vi "BASE-Main.vi"() -> ()   [LabVIEW 2017]
uses:
  <vilib>/Utility/error.llb/DialogType.ctl
panel:
  out "PLC Simulation ON":bool
  in  "Modify SN":bool
  in  "PRINT":bool
  in  "Torque IO Status":bool
  in  "Ass IO Status":bool
  in  "Recipe":bool
  out "error out":errorcluster
  in  "Logout":bool
  in  "Stop":bool
  in  "Create Login":bool
  in  "Reports":bool
  in  "Start":bool
  out "Time":string
  out "Date":string
  in  "Login":bool
  # "KAPSE SONS ROBOTICS\n& AUTOMATION"
  # "RBC TANK"
types:
  T1 = typedef "DialogType.ctl" = u16
  T2 = enum32{"Invalid", "Standard", "Closed", "Hidden", "Minimized", "Maximized"}
  T3 = enum8{"Enabled", "Disabled", "Disabled and Grayed Out"}
  T4 = enum32{"invalid app kind", "Development System", "Run Time System", "Student Edition", "Embedded LabVIEW", "Evaluation", "Custom"}
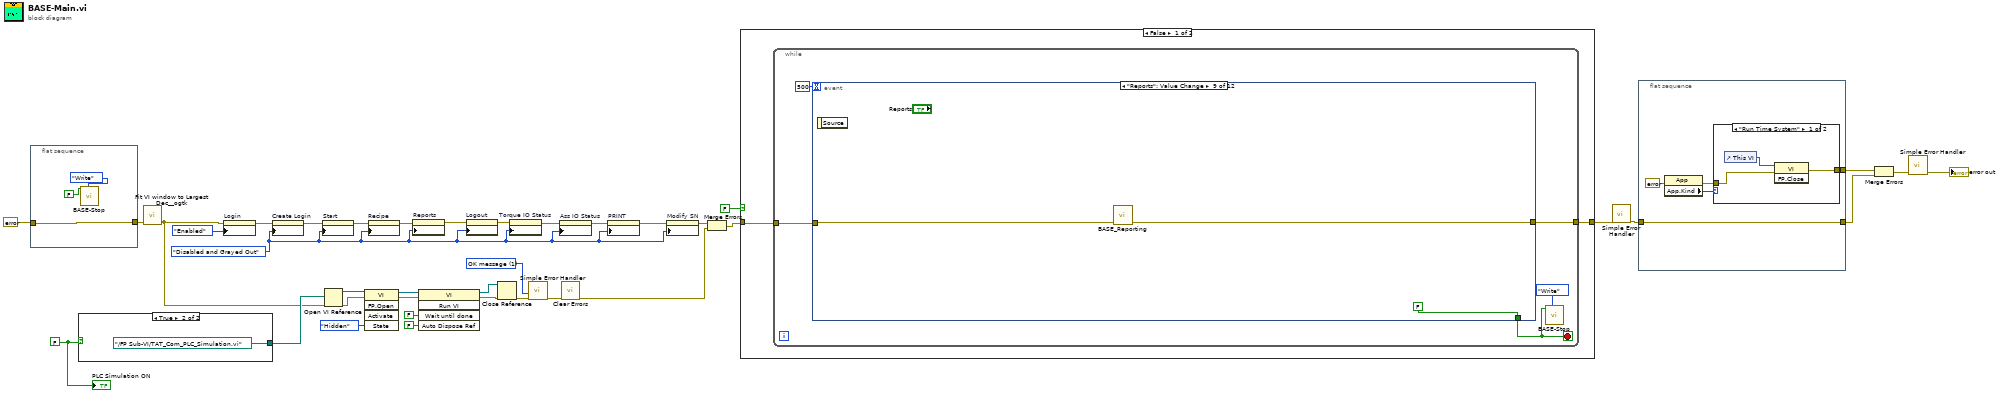
[diagram p0: block diagram]
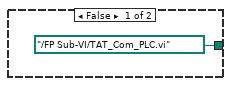
[diagram p2: hidden frame]
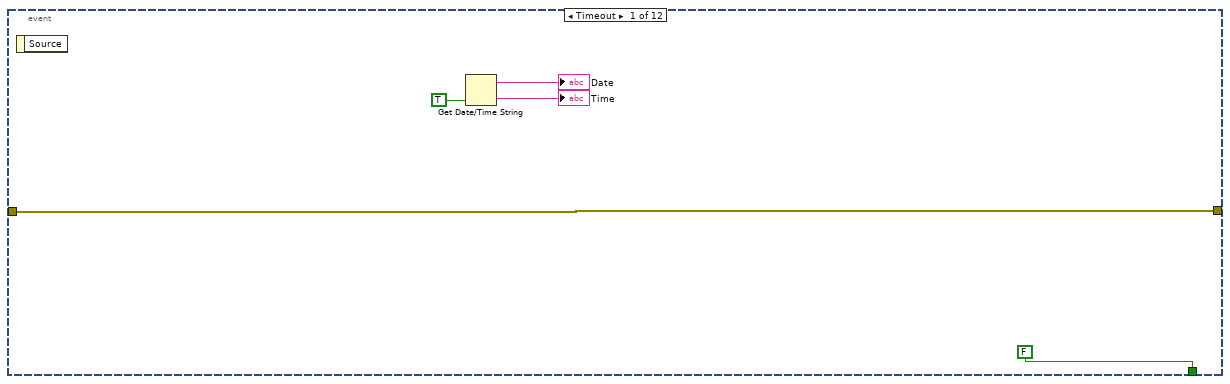
[diagram p4: hidden frame]
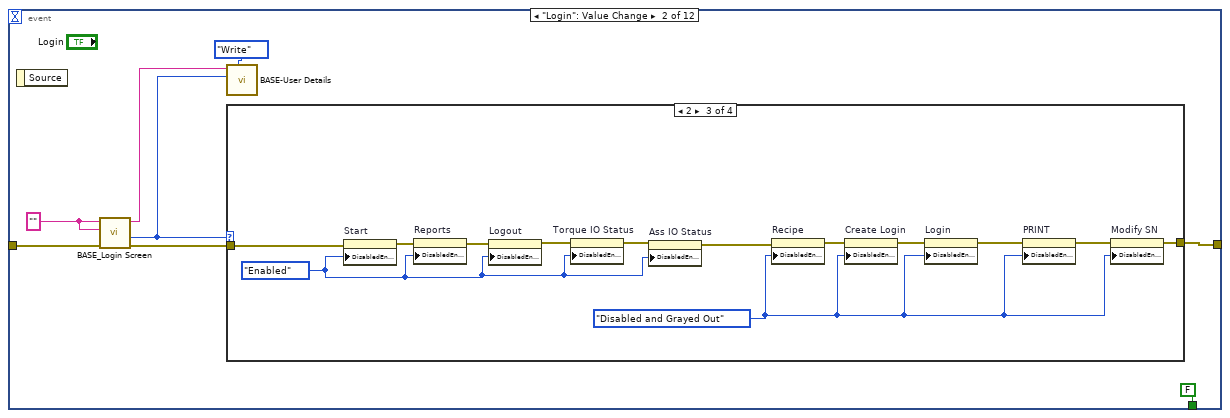
[diagram p5: hidden frame]
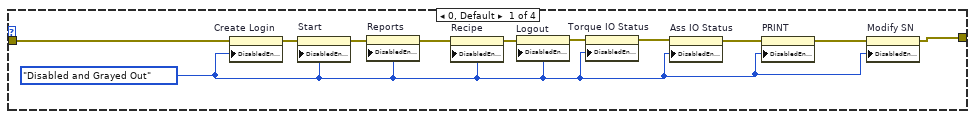
[diagram p6: hidden frame]
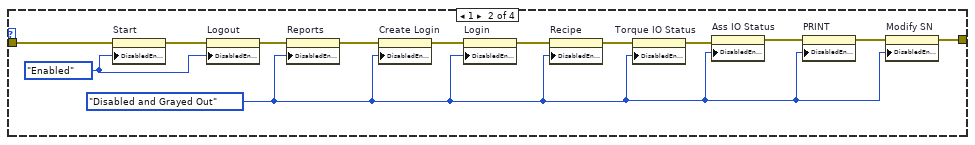
[diagram p7: hidden frame]
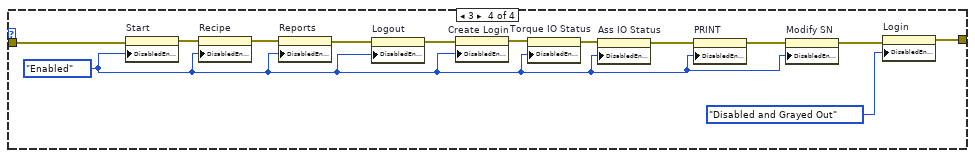
[diagram p8: hidden frame]
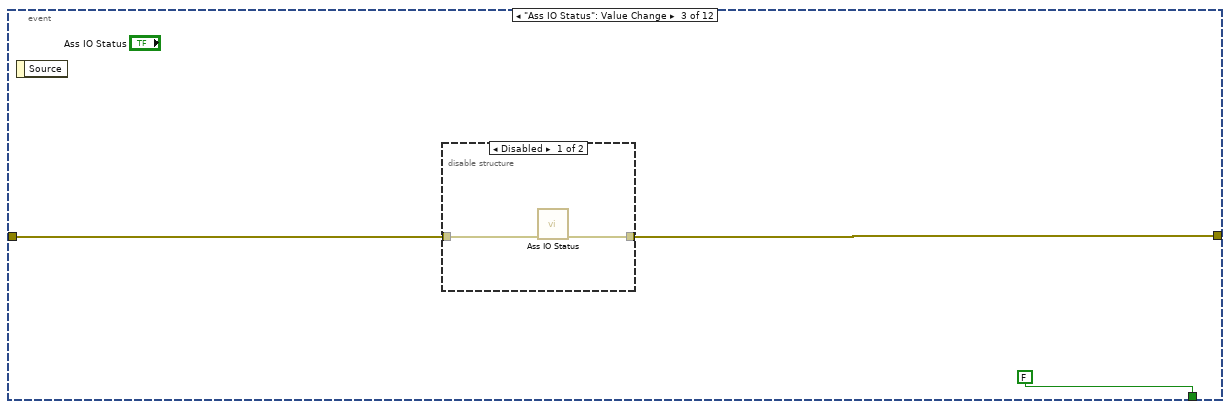
[diagram p9: hidden frame]
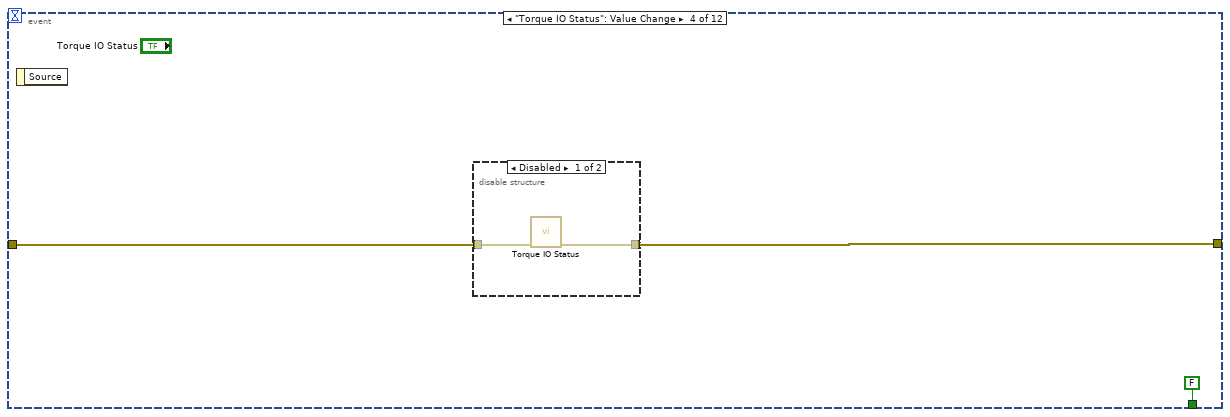
[diagram p11: hidden frame]
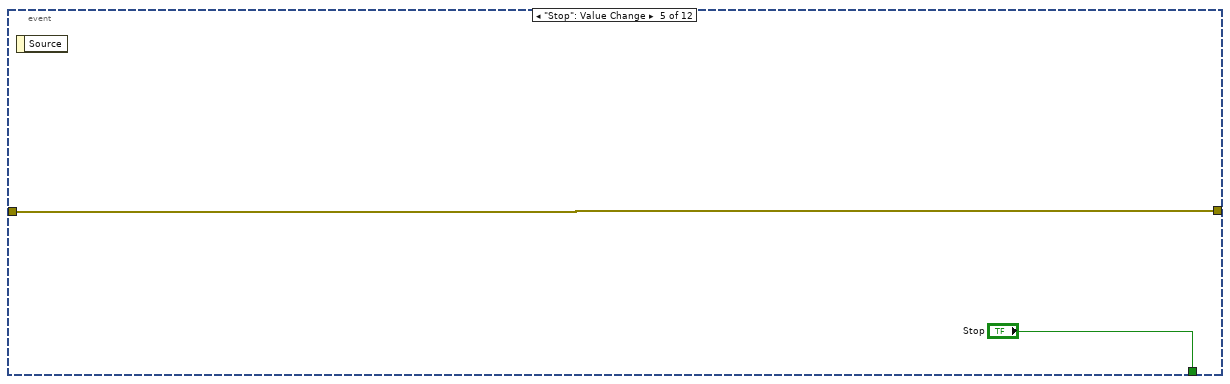
[diagram p13: hidden frame]
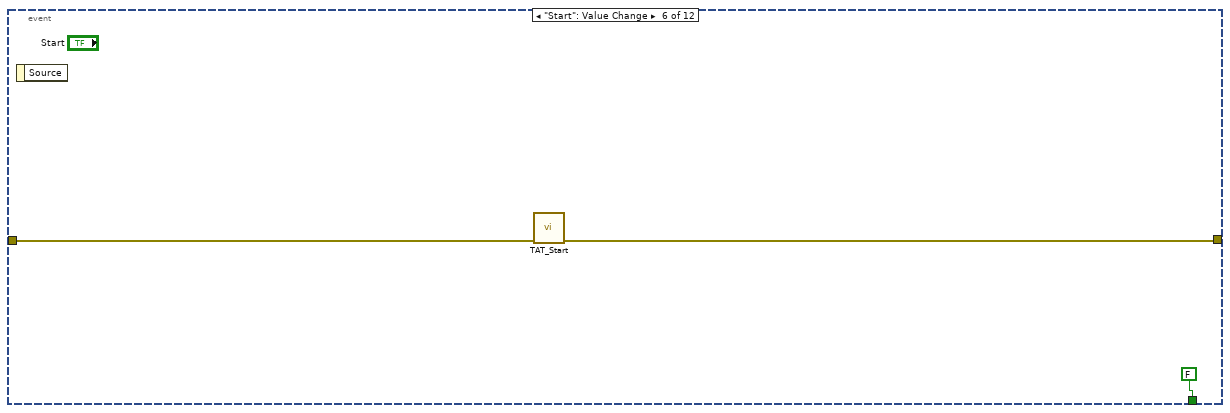
[diagram p14: hidden frame]
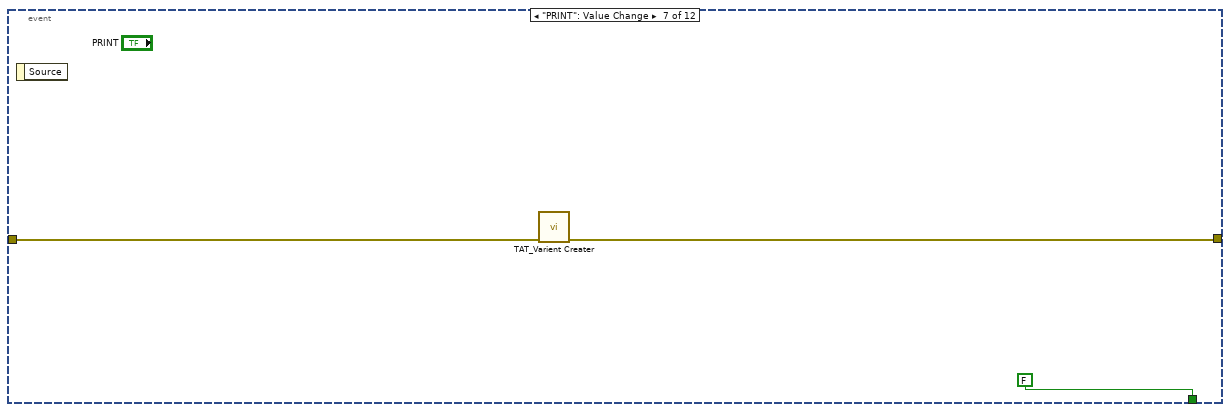
[diagram p15: hidden frame]
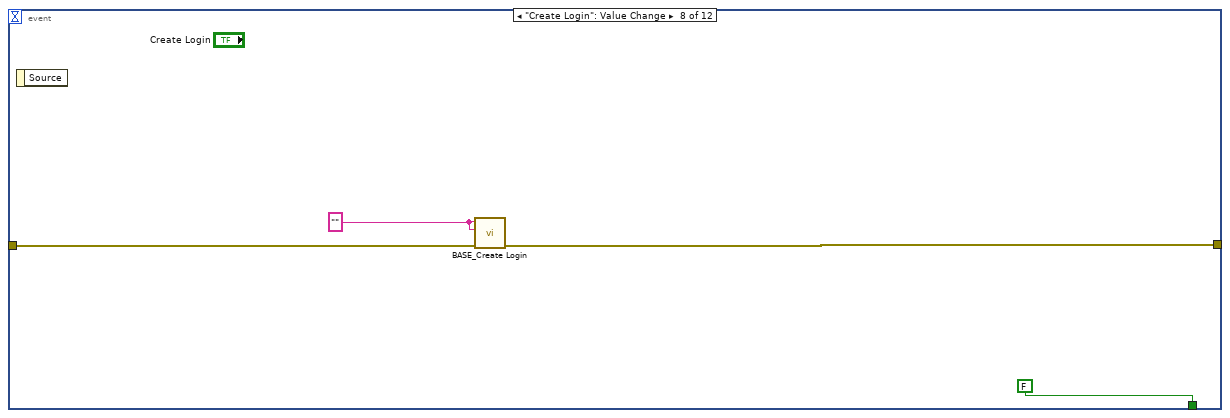
[diagram p16: hidden frame]
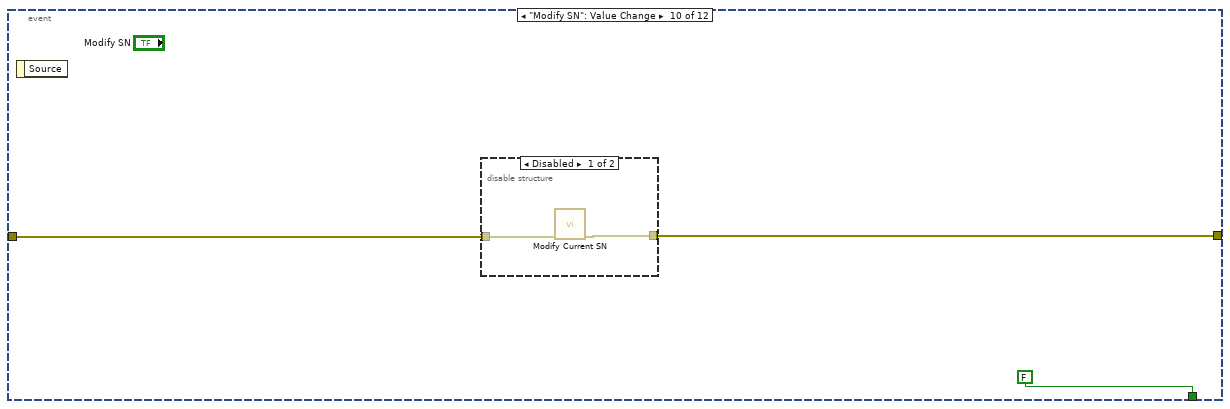
[diagram p17: hidden frame]
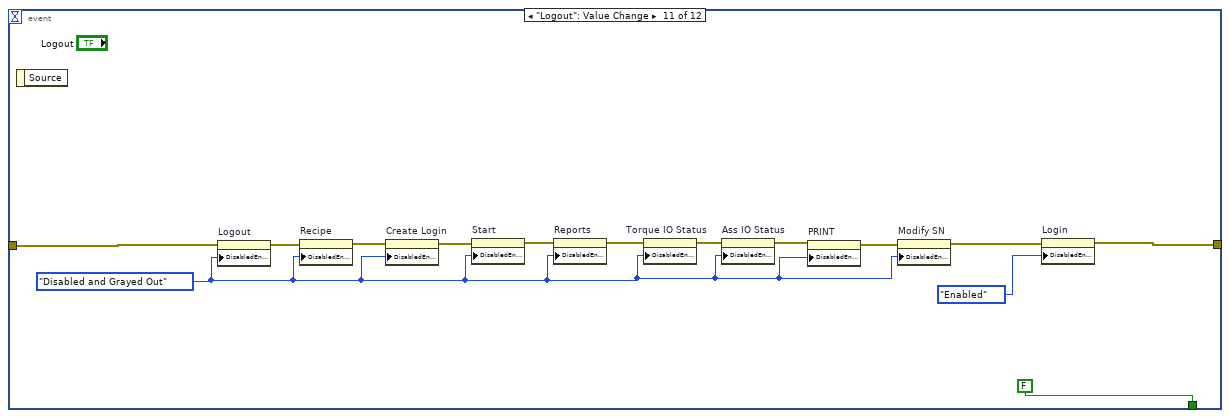
[diagram p19: hidden frame]
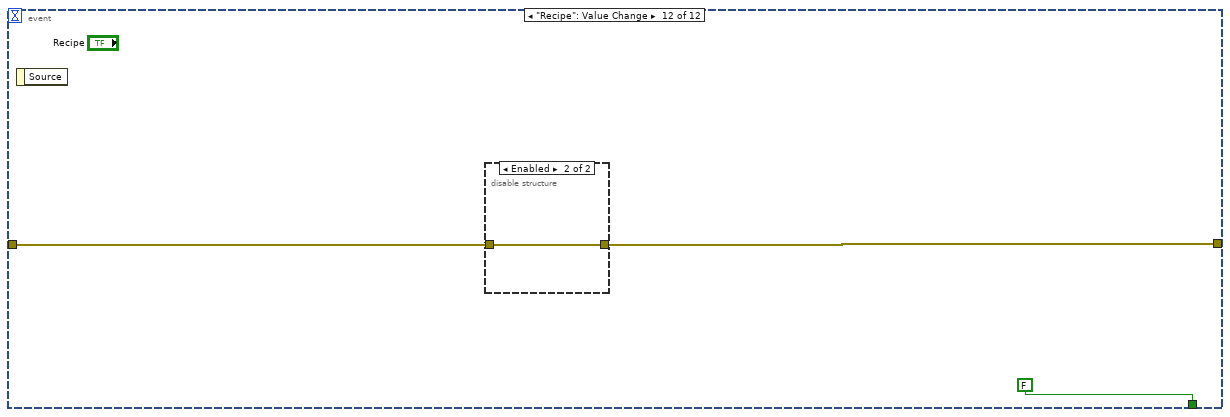
[diagram p20: hidden frame]
diagram:
  w1 = FALSE
  w5 = T1 1 items=["no dialog", "OK message", "continue or stop message", "OK message + warnings", "continue/stop + warnings"] ("type of dialog (OK msg:1)")
  w22 = T3."Disabled and Grayed Out" ("Disabled")
  n1 = flat-sequence {
    tunnel: [w41] -> w20
    tunnel: errorcluster {"status"=FALSE, "code"=0, "source"=""} ("error constant") -> [w41]
    frame #0 {
      n2 = call "BASE-Stop.vi"("Enum"=enum16{"Read", "Write"}."Write", "Stop"=FALSE) -> ()  [unwired: 9 in, 1 out]
    }
  }
  n3 = case shown="True" w1 {
    tunnel: [path "../FP Sub-VI/TAT_Com_PLC.vi" ("vi path") path "../FP Sub-VI/TAT_Com_PLC_Simulation.vi" ("vi path")] -> w11
    frame False {
    }
    frame True {
    }
  }
  n4 = call <userlib>:"Fit VI window to Largest Dec__ogtk.vi"("error in (no error)"=w20) -> ("error out"=w10:errorcluster)  [unwired: 5 in, 1 out]
  n5 = property on="Login" class="Bool"(error in=w10, "DisabledEnum"=T3."Enabled" ("Disabled")) -> (error out=w32:errorcluster)  [unwired: 1 in, 1 out]
  n6 = property on="Create Login" class="Bool"(error in=w32, "DisabledEnum"=w22) -> (error out=w37:errorcluster)  [unwired: 1 in, 1 out]
  n7 = property on="Start" class="Bool"(error in=w37, "DisabledEnum"=w22) -> (error out=w28:errorcluster)  [unwired: 1 in, 1 out]
  n8 = Open VI Reference(vi path=w11, error in (no error)=w10) -> (vi reference=w16:refnum<vi>, error out=w17:errorcluster)  [unwired: 4 in]
  n9 = invoke class="VI" method="FP.Open"(reference=w16, error in=w17, "State"=T2."Hidden") -> (reference out=w19:refnum<vi>, error out=w18:errorcluster)  [unwired: 2 in, 3 out]
  n10 = property on="Recipe" class="Bool"(error in=w28, "DisabledEnum"=w22) -> (error out=w27:errorcluster)  [unwired: 1 in, 1 out]
  n11 = property on="Reports" class="Bool"(error in=w27, "DisabledEnum"=w22) -> (error out=w30:errorcluster)  [unwired: 1 in, 1 out]
  n12 = invoke class="VI" method="Run VI"(reference=w19, error in=w18, "Wait until done"=FALSE ("Wait Until Done"), "Auto Dispose Ref"=FALSE ("Auto Dispose Reference")) -> (reference out=w15:refnum<vi>, error out=w14:errorcluster)  [unwired: 1 in, 3 out]
  n13 = property on="Logout" class="Bool"(error in=w30, "DisabledEnum"=w22) -> (error out=w26:errorcluster)  [unwired: 1 in, 1 out]
  n14 = Close Reference(reference=w15, error in (no error)=w14) -> (error out=w6:errorcluster)
  n15 = property on="Torque IO Status" class="Bool"(error in=w26, "DisabledEnum"=w22) -> (error out=w25:errorcluster)  [unwired: 1 in, 1 out]
  n16 = call <vilib>:"Simple Error Handler.vi"("type of dialog (OK msg:1)"=w5, "error in (no error)"=w6) -> ("error out"=w4:errorcluster)  [unwired: 3 in, 4 out]
  n17 = property on="Ass IO Status" class="Bool"(error in=w25, "DisabledEnum"=w22) -> (error out=w24:errorcluster)  [unwired: 1 in, 1 out]
  n18 = call <vilib>:"Clear Errors.vi"("error in (no error)"=w4) -> ("error out"=w3:errorcluster)  [unwired: 5 in, 1 out]
  n19 = property on="PRINT" class="Bool"(error in=w24, "DisabledEnum"=w22) -> (error out=w23:errorcluster)  [unwired: 1 in, 1 out]
  n20 = property on="Modify SN" class="Bool"(error in=w23, "DisabledEnum"=w22) -> (error out=w8:errorcluster)  [unwired: 1 in, 1 out]
  n21 = Merge Errors(w8, w3) -> (w9:errorcluster)
  n22 = case shown="False" FALSE {
    tunnel: w9 -> [w45 w165]
    tunnel: [w44 w165] -> w38
    frame False {
      n23 = while {
        tunnel: w45 -> [w49]
        tunnel: [w48] -> w44
        stop <- w46 stop-if-true
        n24 = event shown="[8] \"Reports\": Value Change" {
          selector: _ -> [_ _ _ _ _ _ _ _ _ _ _ _]
          dyn-events: _ -> [_ _ _ _ _ _ _ _ _ _ _ _]
          timeout: 500 -> [_ _ _ _ _ _ _ _ _ _ _ _]
          tunnel: w49 -> [w53 w63 w116 w120 w125 w128 w131 w136 w138 w142 w155 w161]
          tunnel: [w53 w61 w115 w119 w125 w127 w130 w135 w137 w141 w156 w160] -> w48
          tunnel: [FALSE ("Stop") FALSE ("Stop") FALSE ("Stop") FALSE ("Stop") "Stop" FALSE ("Stop") FALSE ("Stop") FALSE ("Stop") FALSE ("Stop") FALSE ("Stop") FALSE ("Stop") FALSE ("Stop")] -> w46
          event Timeout {
            n25 = event-data() -> ()  [unwired: 1 in, 1 out]
            n26 = Get Date/Time String(want seconds? (F)=TRUE) -> (date string=→"Date":string, time string=→"Time":string)  [unwired: 2 in]
          }
          event "Login": Value Change {
            w58 = "" ("User Name")
            n27 = event-data() -> ()  [unwired: 1 in, 1 out]
            n28 = call "BASE_Login Screen.vi"("Error In"=w63, "Password"=w58, "User Name"=w58) -> ("error out"=w62:errorcluster, "Level"=w56:i32, "User Name Out"=w59:string)  [unwired: 5 in, 1 out]
            n29 = call "BASE-User Details.vi"("Enum"=enum16{"Read", "Write"}."Write", "Level In"=w56, "User Name In"=w59) -> ()  [unwired: 7 in, 2 out]
            n30 = case shown="2" w56 {
              tunnel: w62 -> [w72 w87 w100 w113]
              tunnel: [w65 w76 w89 w112] -> w61
              frame 0, Default {
                w64 = T3."Disabled and Grayed Out" ("Disabled")
                n31 = property on="Create Login" class="Bool"(error in=w72, "DisabledEnum"=w64) -> (error out=w74:errorcluster)  [unwired: 1 in, 1 out]
                n32 = property on="Start" class="Bool"(error in=w74, "DisabledEnum"=w64) -> (error out=w73:errorcluster)  [unwired: 1 in, 1 out]
                n33 = property on="Reports" class="Bool"(error in=w73, "DisabledEnum"=w64) -> (error out=w71:errorcluster)  [unwired: 1 in, 1 out]
                n34 = property on="Recipe" class="Bool"(error in=w71, "DisabledEnum"=w64) -> (error out=w70:errorcluster)  [unwired: 1 in, 1 out]
                n35 = property on="Logout" class="Bool"(error in=w70, "DisabledEnum"=w64) -> (error out=w69:errorcluster)  [unwired: 1 in, 1 out]
                n36 = property on="Torque IO Status" class="Bool"(error in=w69, "DisabledEnum"=w64) -> (error out=w68:errorcluster)  [unwired: 1 in, 1 out]
                n37 = property on="Ass IO Status" class="Bool"(error in=w68, "DisabledEnum"=w64) -> (error out=w67:errorcluster)  [unwired: 1 in, 1 out]
                n38 = property on="PRINT" class="Bool"(error in=w67, "DisabledEnum"=w64) -> (error out=w66:errorcluster)  [unwired: 1 in, 1 out]
                n39 = property on="Modify SN" class="Bool"(error in=w66, "DisabledEnum"=w64) -> (error out=w65:errorcluster)  [unwired: 1 in, 1 out]
              }
              frame 1 {
                w75 = T3."Disabled and Grayed Out" ("Disabled")
                w83 = T3."Enabled" ("Disabled")
                n40 = property on="Start" class="Bool"(error in=w87, "DisabledEnum"=w83) -> (error out=w82:errorcluster)  [unwired: 1 in, 1 out]
                n41 = property on="Logout" class="Bool"(error in=w82, "DisabledEnum"=w83) -> (error out=w85:errorcluster)  [unwired: 1 in, 1 out]
                n42 = property on="Reports" class="Bool"(error in=w85, "DisabledEnum"=w75) -> (error out=w86:errorcluster)  [unwired: 1 in, 1 out]
                n43 = property on="Create Login" class="Bool"(error in=w86, "DisabledEnum"=w75) -> (error out=w84:errorcluster)  [unwired: 1 in, 1 out]
                n44 = property on="Login" class="Bool"(error in=w84, "DisabledEnum"=w75) -> (error out=w81:errorcluster)  [unwired: 1 in, 1 out]
                n45 = property on="Recipe" class="Bool"(error in=w81, "DisabledEnum"=w75) -> (error out=w79:errorcluster)  [unwired: 1 in, 1 out]
                n46 = property on="Torque IO Status" class="Bool"(error in=w79, "DisabledEnum"=w75) -> (error out=w80:errorcluster)  [unwired: 1 in, 1 out]
                n47 = property on="Ass IO Status" class="Bool"(error in=w80, "DisabledEnum"=w75) -> (error out=w78:errorcluster)  [unwired: 1 in, 1 out]
                n48 = property on="PRINT" class="Bool"(error in=w78, "DisabledEnum"=w75) -> (error out=w77:errorcluster)  [unwired: 1 in, 1 out]
                n49 = property on="Modify SN" class="Bool"(error in=w77, "DisabledEnum"=w75) -> (error out=w76:errorcluster)  [unwired: 1 in, 1 out]
              }
              frame 2 {
                w88 = T3."Disabled and Grayed Out" ("Disabled")
                w92 = T3."Enabled" ("Disabled")
                n50 = property on="Start" class="Bool"(error in=w100, "DisabledEnum"=w92) -> (error out=w97:errorcluster)  [unwired: 1 in, 1 out]
                n51 = property on="Reports" class="Bool"(error in=w97, "DisabledEnum"=w92) -> (error out=w99:errorcluster)  [unwired: 1 in, 1 out]
                n52 = property on="Logout" class="Bool"(error in=w99, "DisabledEnum"=w92) -> (error out=w94:errorcluster)  [unwired: 1 in, 1 out]
                n53 = property on="Torque IO Status" class="Bool"(error in=w94, "DisabledEnum"=w92) -> (error out=w95:errorcluster)  [unwired: 1 in, 1 out]
                n54 = property on="Ass IO Status" class="Bool"(error in=w95, "DisabledEnum"=w92) -> (error out=w93:errorcluster)  [unwired: 1 in, 1 out]
                n55 = property on="Recipe" class="Bool"(error in=w93, "DisabledEnum"=w88) -> (error out=w96:errorcluster)  [unwired: 1 in, 1 out]
                n56 = property on="Create Login" class="Bool"(error in=w96, "DisabledEnum"=w88) -> (error out=w98:errorcluster)  [unwired: 1 in, 1 out]
                n57 = property on="Login" class="Bool"(error in=w98, "DisabledEnum"=w88) -> (error out=w91:errorcluster)  [unwired: 1 in, 1 out]
                n58 = property on="PRINT" class="Bool"(error in=w91, "DisabledEnum"=w88) -> (error out=w90:errorcluster)  [unwired: 1 in, 1 out]
                n59 = property on="Modify SN" class="Bool"(error in=w90, "DisabledEnum"=w88) -> (error out=w89:errorcluster)  [unwired: 1 in, 1 out]
              }
              frame 3 {
                w101 = T3."Enabled" ("Disabled")
                n60 = property on="Start" class="Bool"(error in=w113, "DisabledEnum"=w101) -> (error out=w108:errorcluster)  [unwired: 1 in, 1 out]
                n61 = property on="Recipe" class="Bool"(error in=w108, "DisabledEnum"=w101) -> (error out=w107:errorcluster)  [unwired: 1 in, 1 out]
                n62 = property on="Reports" class="Bool"(error in=w107, "DisabledEnum"=w101) -> (error out=w110:errorcluster)  [unwired: 1 in, 1 out]
                n63 = property on="Logout" class="Bool"(error in=w110, "DisabledEnum"=w101) -> (error out=w109:errorcluster)  [unwired: 1 in, 1 out]
                n64 = property on="Create Login" class="Bool"(error in=w109, "DisabledEnum"=w101) -> (error out=w106:errorcluster)  [unwired: 1 in, 1 out]
                n65 = property on="Torque IO Status" class="Bool"(error in=w106, "DisabledEnum"=w101) -> (error out=w105:errorcluster)  [unwired: 1 in, 1 out]
                n66 = property on="Ass IO Status" class="Bool"(error in=w105, "DisabledEnum"=w101) -> (error out=w104:errorcluster)  [unwired: 1 in, 1 out]
                n67 = property on="PRINT" class="Bool"(error in=w104, "DisabledEnum"=w101) -> (error out=w103:errorcluster)  [unwired: 1 in, 1 out]
                n68 = property on="Modify SN" class="Bool"(error in=w103, "DisabledEnum"=w101) -> (error out=w102:errorcluster)  [unwired: 1 in, 1 out]
                n69 = property on="Login" class="Bool"(error in=w102, "DisabledEnum"=T3."Disabled and Grayed Out" ("Disabled")) -> (error out=w112:errorcluster)  [unwired: 1 in, 1 out]
              }
            }
          }
          event "Ass IO Status": Value Change {
            n70 = event-data() -> ()  [unwired: 1 in, 1 out]
            n71 = disable-structure shown="Disabled" {
              disable-tunnel: w116 -> [w118 _]
              disable-tunnel: [w117 _] -> w115
              frame Disabled {
                n72 = call "Ass IO Status.vi"("error in (no error)"=w118) -> ("error out"=w117:errorcluster)  [unwired: 10 in]
              }
              frame Enabled {
              }
            }
          }
          event "Torque IO Status": Value Change {
            n73 = event-data() -> ()  [unwired: 1 in, 1 out]
            n74 = disable-structure shown="Disabled" {
              disable-tunnel: w120 -> [w123 w124]
              disable-tunnel: [w122 w124] -> w119
              frame Disabled {
                n75 = call "Torque IO Status.vi"("error in (no error)"=w123) -> ("error out"=w122:errorcluster)  [unwired: 10 in]
              }
              frame Enabled {
              }
            }
          }
          event "Stop": Value Change {
            n76 = event-data() -> ()  [unwired: 1 in, 1 out]
          }
          event "Start": Value Change {
            n77 = event-data() -> ()  [unwired: 1 in, 1 out]
            n78 = call "TAT_Start.vi"("error In"=w128) -> ("error out"=w127:errorcluster)  [unwired: 10 in]
          }
          event "PRINT": Value Change {
            n79 = event-data() -> ()  [unwired: 1 in, 1 out]
            n80 = call "TAT_Varient Creater.vi"("error in (no error)"=w131) -> ("error out"=w130:errorcluster)  [unwired: 10 in]
          }
          event "Create Login": Value Change {
            w134 = "" ("User Name")
            n81 = event-data() -> ()  [unwired: 1 in, 1 out]
            n82 = call "BASE_Create Login.vi"("Error In"=w136, "Password"=w134, "User Name"=w134) -> ("error out"=w135:errorcluster)  [unwired: 6 in]
          }
          event "Reports": Value Change {
            n83 = event-data() -> ()  [unwired: 1 in, 1 out]
            n84 = call "BASE_Reporting.vi"("error in (no error)"=w138) -> ("error out"=w137:errorcluster)  [unwired: 10 in]
          }
          event "Modify SN": Value Change {
            n85 = event-data() -> ()  [unwired: 1 in, 1 out]
            n86 = disable-structure shown="Disabled" {
              disable-tunnel: w142 -> [w144 _]
              disable-tunnel: [w143 _] -> w141
              frame Disabled {
                n87 = call "Modify Current SN.vi"("error in (no error)"=w144) -> ("error out"=w143:errorcluster)  [unwired: 10 in]
              }
              frame Enabled {
              }
            }
          }
          event "Logout": Value Change {
            w145 = T3."Disabled and Grayed Out" ("Disabled")
            n88 = event-data() -> ()  [unwired: 1 in, 1 out]
            n89 = property on="Logout" class="Bool"(error in=w155, "DisabledEnum"=w145) -> (error out=w153:errorcluster)  [unwired: 1 in, 1 out]
            n90 = property on="Recipe" class="Bool"(error in=w153, "DisabledEnum"=w145) -> (error out=w152:errorcluster)  [unwired: 1 in, 1 out]
            n91 = property on="Create Login" class="Bool"(error in=w152, "DisabledEnum"=w145) -> (error out=w158:errorcluster)  [unwired: 1 in, 1 out]
            n92 = property on="Start" class="Bool"(error in=w158, "DisabledEnum"=w145) -> (error out=w157:errorcluster)  [unwired: 1 in, 1 out]
            n93 = property on="Reports" class="Bool"(error in=w157, "DisabledEnum"=w145) -> (error out=w150:errorcluster)  [unwired: 1 in, 1 out]
            n94 = property on="Torque IO Status" class="Bool"(error in=w150, "DisabledEnum"=w145) -> (error out=w151:errorcluster)  [unwired: 1 in, 1 out]
            n95 = property on="Ass IO Status" class="Bool"(error in=w151, "DisabledEnum"=w145) -> (error out=w148:errorcluster)  [unwired: 1 in, 1 out]
            n96 = property on="PRINT" class="Bool"(error in=w148, "DisabledEnum"=w145) -> (error out=w147:errorcluster)  [unwired: 1 in, 1 out]
            n97 = property on="Modify SN" class="Bool"(error in=w147, "DisabledEnum"=w145) -> (error out=w146:errorcluster)  [unwired: 1 in, 1 out]
            n98 = property on="Login" class="Bool"(error in=w146, "DisabledEnum"=T3."Enabled" ("Disabled")) -> (error out=w156:errorcluster)  [unwired: 1 in, 1 out]
          }
          event "Recipe": Value Change {
            n99 = event-data() -> ()  [unwired: 1 in, 1 out]
            n100 = disable-structure shown="Enabled" {
              disable-tunnel: w161 -> [w163 w164]
              disable-tunnel: [w162 w164] -> w160
              frame Disabled {
                n101 = call "TAT-Create Reciepe.vi"("Error In"=w163) -> ("error out"=w162:errorcluster)  [unwired: 10 in]
              }
              frame Enabled {
              }
            }
          }
        }
        n102 = call "BASE-Stop.vi"("Enum"=enum16{"Read", "Write"}."Write", "Stop"=w46) -> ()  [unwired: 9 in, 1 out]
      }
    }
    frame True {
    }
  }
  n103 = call <vilib>:"Simple Error Handler.vi"("error in (no error)"=w38) -> ("error out"=w33:errorcluster)  [unwired: 4 in, 4 out]
  n104 = flat-sequence {
    tunnel: [w167] -> w36
    tunnel: [w166] -> w34
    tunnel: w33 -> [w166]
    frame #0 {
      n105 = property class="App"(error in=errorcluster {"status"=FALSE, "code"=0, "source"=""} ("error in (no error)")) -> (error out=w169:errorcluster, "App.Kind"=w170:T4)  [unwired: 1 in, 1 out]
      n106 = case shown="\"Run Time System\"" w170 {
        tunnel: w169 -> [w172 w174]
        tunnel: [w171 w174] -> w167
        frame "Run Time System" {
          n107 = control-ref of="This VI"() -> (w173:refnum<vi>)
          n108 = invoke class="VI" method="FP.Close"(reference=w173, error in=w172) -> (error out=w171:errorcluster)  [unwired: 1 in, 2 out]
        }
        frame "Development System", Default {
        }
      }
    }
  }
  n109 = Merge Errors(w36, w34) -> (w35:errorcluster)
  n110 = call <vilib>:"Simple Error Handler.vi"("error in (no error)"=w35) -> ("error out"=→"error out":errorcluster)  [unwired: 4 in, 4 out]
  "PLC Simulation ON" <- w1
